vi "Handle.vi"(11 "Base Event Actor in":refnum<class "Base Event Actor.lvclass">) -> (2 "Destroy?":bool, 3 "Base Event Actor out":refnum<class "Base Event Actor.lvclass">)   [LabVIEW 2021, in "jettl.lvlib" / "Base Event Actor.lvclass"]
uses:
  Base Event Actor.lvclass
  C:/git/jettl/src/jettl/Event Actor/Event Actor.lvclass
  Base Event Actor.lvclass/Base Event Actor.ctl
  Event State/Event State/Event State.lvclass
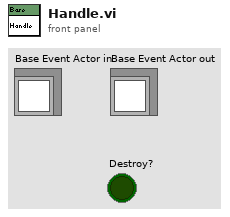
[diagram p1: front panel]
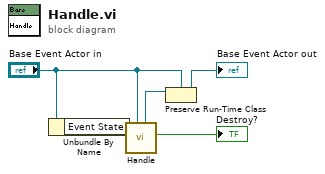
[diagram p0: block diagram]
diagram:
  n1 = Unbundle By Name("Base Event Actor in") -> ("Event State"=w4:refnum<class "Event State.lvclass">)
  n2 = call-dynamic "Handle.vi"("Event Actor in"="Base Event Actor in", "Event State in"=w4) -> ("Destroy?"=→"Destroy?":bool, "Event Actor out"=w2:refnum<class "Event Actor.lvclass">)  [unwired: 8 in]
  n3 = Preserve Run-Time Class(object in=w2, 2:"Base Event Actor in") -> (object out=→"Base Event Actor out":refnum<class "Base Event Actor.lvclass">)  [unwired: 1 in, 1 out]
